vi "Enqueue Signal.vi"(0 "reference in":refnum<class "Logger.lvclass">, 5 "element":T1, 11 "error in (no error)":errorcluster) -> (4 "reference out":refnum<class "Logger.lvclass">, 15 "error out":errorcluster)   [LabVIEW 2019, in "Logger.lvclass"]
uses:
  Logger.lvclass
  SignalData.ctl
  Logger.lvclass/Logger.ctl
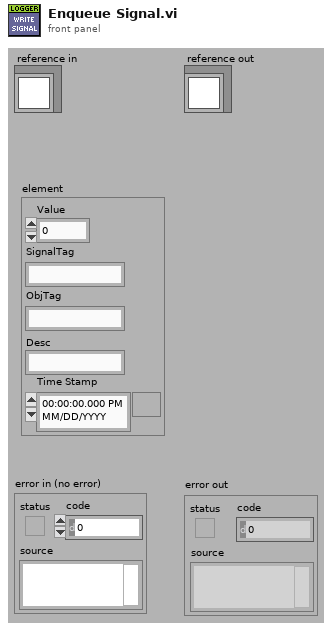
[diagram p1: front panel]
types:
  T1 = typedef "Logger.lvclass/SignalData.ctl" = cluster{"Value":dbl, "SignalTag":string, "ObjTag":string, "Desc":string, "Time Stamp":timestamp}
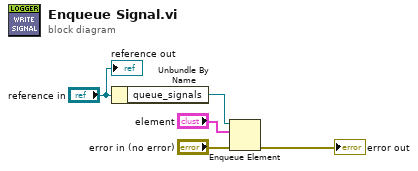
[diagram p0: block diagram]
diagram:
  n1 = Unbundle By Name("reference in") -> ("queue_signals"=w1:refnum<queue>)
  n2 = Enqueue Element(queue=w1, element="element", error in (no error)="error in (no error)") -> (error out=→"error out":errorcluster)  [unwired: 1 in, 2 out]
  "reference out" <- "reference in"
